vi "Module (Rename).vi"(8 "Error In":errorcluster) -> (0 "Last Error":errorcluster)   [LabVIEW 2015, in "Generic Module Library.lvlib" / "Template G_Module.lvlib"]
uses:
  Template G_Module.lvlib
  Module Class/Rename.lvclass
panel:
  in  "Stop":bool
  in  "Debug Toggle":bool
  in  "Debug Tab":T1(tab)
  out "Timing Target (ms)":i16
  out "Module Iterations":u64
  out "Last Executed Case":string
  in  "Configure":bool
  in  "View Log":bool
  in  "Ping":bool
  out "Ping Response":string
  out "Debug Log":string
  out "Received @":timestamp
  out "Current Error":errorcluster
  out "Received @":timestamp
  out "Received @":timestamp
  # ">>Newest>>"
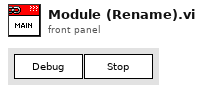
[diagram p1: front panel]
types:
  T1 = enum32{"Module Data/Commands", "Module Log", "Current Error", "Start Error", "Close Error"}
  T2 = typedef "Generic Module Library.lvlib/Template G_Module.lvlib/Broadcast List.ctl" = cluster{"Module Started":refnum<user-event>, "Module Error":refnum<user-event>, "Module Pong":refnum<user-event>, "Module Status":refnum<user-event>, "Module Stopping":refnum<user-event>, "Module Stopped":refnum<user-event>, "Module Reinitialized":refnum<user-event>}
  T3 = cluster{"Event Registration Refnum":refnum<event-registration>, "Stop Event Refnum":refnum<event-registration>}
  T4 = typedef "Generic Module Library.lvlib/Template G_Module.lvlib/Acknowledge Data Cluster.ctl" = cluster{"Ack Requested":bool, "Ack Notifier Ref":refnum<notifier>, "Response Payload":T5}
  T5 = typedef "Generic Module Library.lvlib/Template G_Module.lvlib/Ack Payload.ctl" = cluster{"Response Data":string, "error out":errorcluster}
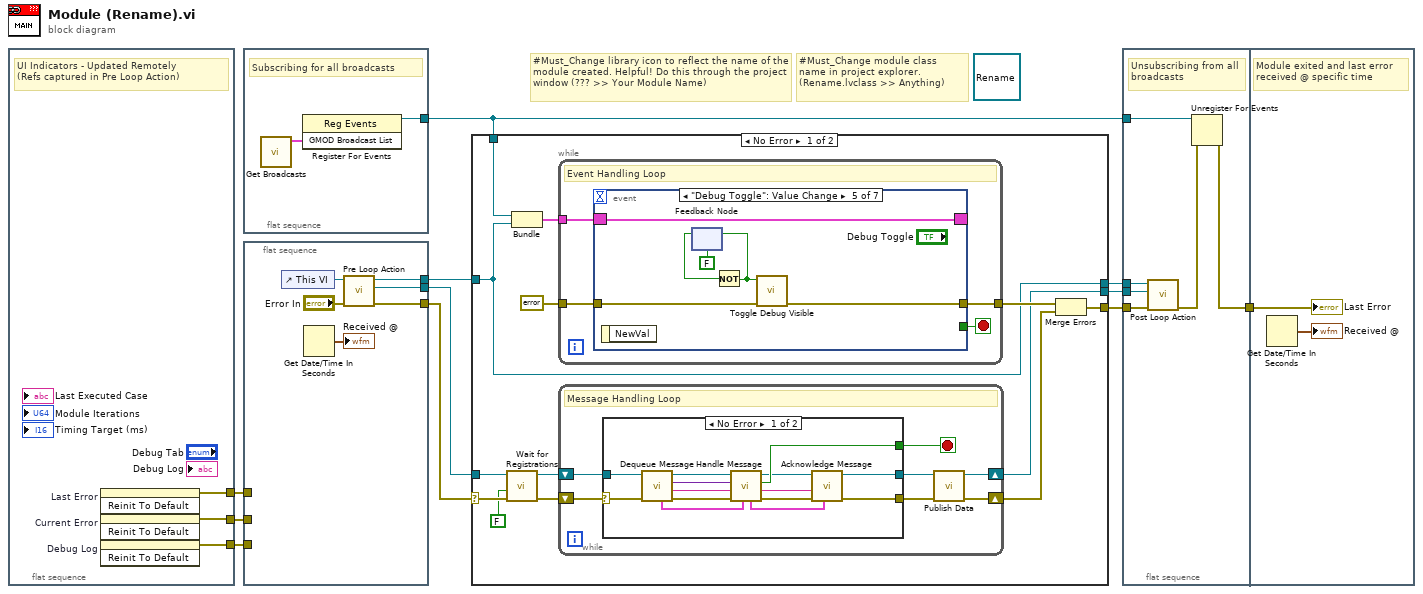
[diagram p0: block diagram]
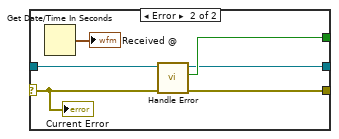
[diagram p2: hidden frame]
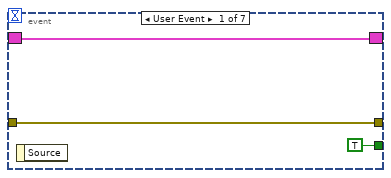
[diagram p3: hidden frame]
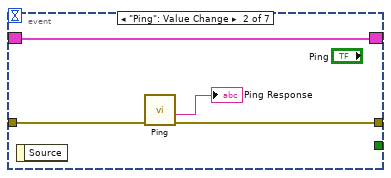
[diagram p4: hidden frame]
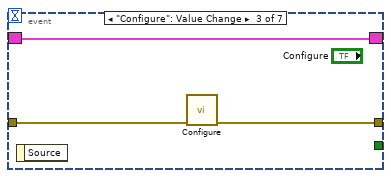
[diagram p5: hidden frame]
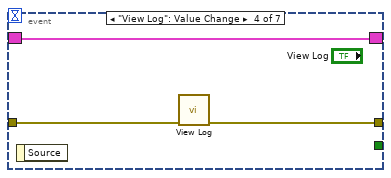
[diagram p6: hidden frame]
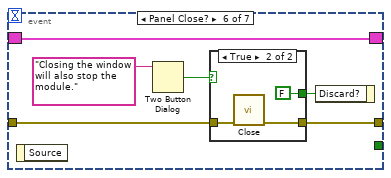
[diagram p7: hidden frame]
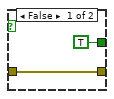
[diagram p8: hidden frame]
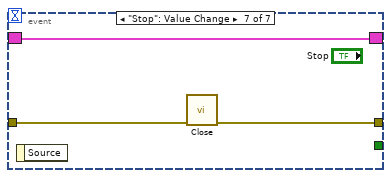
[diagram p9: hidden frame]
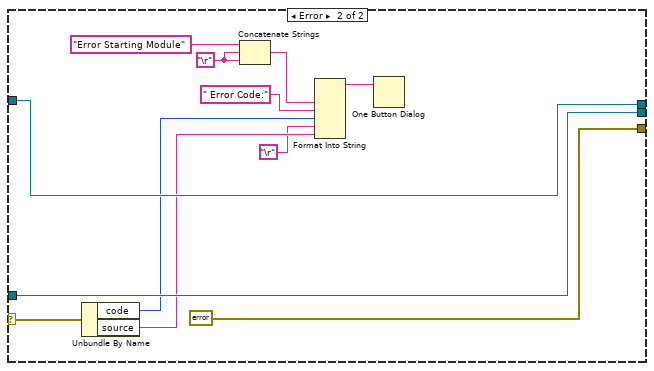
[diagram p10: hidden frame]
diagram:
  (unwired) refnum<class "Rename.lvclass"> refnum ("Generic Module Library.lvlib:Template G_Module.lvlib:Rename.lvclass")
  # "#Must_Change library icon to reflect the name of the module created. Helpful! Do this through the project window (??? >> Your Module Name)"
  # "#Must_Change module class name in project explorer. (Rename.lvclass >> Anything)"
  n1 = flat-sequence {
    tunnel: [w14] -> w5
    tunnel: [w13] -> w4
    tunnel: [w12] -> w3
    frame #0 {
      # "UI Indicators - Updated Remotely \n(Refs captured in Pre Loop Action)"
      n2 = invoke on="Last Error" class="Clust (strict)" method="Reinit To Default"() -> (error out=w14:errorcluster)  [unwired: 3 in, 2 out]
      n3 = invoke on="Current Error" class="Clust (strict)" method="Reinit To Default"() -> (error out=w13:errorcluster)  [unwired: 3 in, 2 out]
      n4 = invoke on="Debug Log" class="Str" method="Reinit To Default"() -> (error out=w12:errorcluster)  [unwired: 3 in, 2 out]
    }
  }
  n5 = flat-sequence {
    tunnel: [w15] -> w2
    frame #0 {
      # "Subscribing for all broadcasts"
      n6 = call "Get Broadcasts.vi"() -> ("GMOD Broadcast List"=w16:T2)  [unwired: 9 in, 2 out]
      n7 = register-events(w16) -> (reference out=w15:refnum<event-registration>)  [unwired: 2 in, 1 out]
    }
  }
  n8 = flat-sequence {
    tunnel: [w19] -> w11
    tunnel: [w18] -> w1
    tunnel: [w17] -> w6
    tunnel: w5 -> [_]
    tunnel: w4 -> [_]
    tunnel: w3 -> [_]
    frame #0 {
      n9 = control-ref of="This VI"() -> (w22:refnum<vi>)
      n10 = Get Date/Time In Seconds() -> (seconds since 1Jan1904=→"Received @":timestamp)
      n11 = call "Pre Loop Action.vi"("error in"="Error In", "Ref In"=w22) -> ("error out"=w17:errorcluster, "Module Data Out"=w19:refnum<class "Rename.lvclass">, "Stop Event Refnum"=w18:refnum<event-registration>)  [unwired: 7 in]
    }
  }
  n12 = case shown="No Error" w6 {
    selector: w6 -> [w27 w103]
    tunnel: w11 -> [w34 w111]
    tunnel: [w32 errorcluster {"status"=FALSE, "code"=0, "source"=""} ("error IO")] -> w9
    tunnel: [w31 w111] -> w8
    tunnel: [w23 w110] -> w7
    tunnel: w2 -> [w25 _]
    tunnel: w1 -> [w23 w110]
    frame No Error {
      n13 = call "Wait for Registrations.vi"("error in"=w27, "Wait for Reg Confirmation? (F)"=FALSE, "Module Data In"=w34) -> ("error out"=w29:errorcluster, "Module Data Out"=w30:refnum<class "Rename.lvclass">)  [unwired: 6 in, 1 out]
      n14 = Bundle("Event Registration Refnum"=w25, "Stop Event Refnum"=w23) -> (w24:T3)  [unwired: 1 in]
      n15 = while {
        tunnel: w24 -> [w64]
        tunnel: errorcluster {"status"=FALSE, "code"=0, "source"=""} ("error out") -> [w65]
        tunnel: [w66] -> w35
        stop <- w63 stop-if-true
        # "Event Handling Loop"
        n16 = event shown="[4] \"Debug Toggle\": Value Change" {
          selector: w64 -> [w67 w70 w76 w79 w85 w86 w99]
          dyn-events: [w67 w70 w76 w79 w85 w86 w99] -> _
          timeout: _ -> [_ _ _ _ _ _ _]
          tunnel: [w69 w72 w74 w77 w83 w89 w97] -> w66
          tunnel: w65 -> [w69 w73 w75 w78 w84 w90 w98]
          tunnel: [TRUE _ _ _ _ _ _] -> w63
          event User Event {
            n17 = event-data() -> ()  [unwired: 1 in, 1 out]
          }
          event "Ping": Value Change {
            n18 = event-data() -> ()  [unwired: 1 in, 1 out]
            n19 = call "Ping.vi"("error in"=w73) -> ("error out"=w72:errorcluster, "Response"=→"Ping Response":string)  [unwired: 8 in, 1 out]
          }
          event "Configure": Value Change {
            n20 = event-data() -> ()  [unwired: 1 in, 1 out]
            n21 = call "Configure.vi"("error in"=w75) -> ("error out"=w74:errorcluster)  [unwired: 10 in]
          }
          event "View Log": Value Change {
            n22 = event-data() -> ()  [unwired: 1 in, 1 out]
            n23 = call "View Log.vi"("error in"=w78) -> ("error out"=w77:errorcluster)  [unwired: 10 in]
          }
          event "Debug Toggle": Value Change {
            n24 = event-data() -> ()  [unwired: 1 in, 1 out]
            n25 = feedback #1(FALSE) -> (w81:bool)
            n26 = Not(x=w81) -> (.not. x?=w82:bool)
            n27 = feedback-in #1(w82) -> ()
            n28 = call "Toggle Debug Visible.vi"("error in"=w84, "Visible?"=w82) -> ("error out"=w83:errorcluster)  [unwired: 9 in]
          }
          event Panel Close? {
            n29 = event-data() -> ()  [unwired: 1 in, 1 out]
            n30 = Two Button Dialog(message="Closing the window will also stop the module.") -> (T button?=w87:bool)  [unwired: 2 in]
            n31 = case shown="True" w87 {
              tunnel: [TRUE ("Discard?") FALSE ("Discard?")] -> w91
              tunnel: w90 -> [w92 w95]
              tunnel: [w92 w94] -> w89
              frame False {
              }
              frame True {
                n32 = call "Close.vi"("error in"=w95) -> ("error out"=w94:errorcluster)  [unwired: 9 in, 1 out]
              }
            }
            n33 = event-data("Discard?"=w91) -> ()  [unwired: 1 in, 1 out]
          }
          event "Stop": Value Change {
            n34 = event-data() -> ()  [unwired: 1 in, 1 out]
            n35 = call "Close.vi"("error in"=w98) -> ("error out"=w97:errorcluster)  [unwired: 9 in, 1 out]
          }
        }
      }
      n36 = while {
        shift-right: [w36] -> w31
        shift-left: w30 -> [w41]
        shift-right: [w37] -> w33
        shift-left: w29 -> [w40]
        stop <- w42 stop-if-true
        # "Message Handling Loop"
        n37 = case shown="No Error" w40 {
          selector: w40 -> [w55 w57]
          tunnel: [w50 w62] -> w42
          tunnel: [w54 w61] -> w39
          tunnel: [w53 w60] -> w38
          tunnel: w41 -> [w56 w59]
          frame No Error {
            n38 = call "Dequeue Message.vi"("error in"=w55, "Module Data In"=w56) -> ("error out"=w46:errorcluster, "Module Action"=w45:string, "Message Data"=w44:variant, "Module Data Out"=w43:refnum<class "Rename.lvclass">, "Acknowledge Data"=w47:T4)  [unwired: 5 in]
            n39 = call "Handle Message.vi"("Acknowledge Data"=w47, "error in (no error)"=w46, "Module Action"=w45, "Message Data Out"=w44, "Module Data In"=w43) -> ("error out"=w52:errorcluster, "Module Action"=w51:string, "Stop Module"=w50:bool, "Module Data Out"=w49:refnum<class "Rename.lvclass">, "Acknowledge Data"=w48:T4)  [unwired: 2 in]
            n40 = call "Acknowledge Message.vi"("Acknowledge Data"=w48, "error in"=w52, "Module Action"=w51, "Module Data In"=w49) -> ("error out"=w54:errorcluster, "Module Data Out"=w53:refnum<class "Rename.lvclass">)  [unwired: 6 in]
          }
          frame Error {
            n41 = Get Date/Time In Seconds() -> (seconds since 1Jan1904=→"Received @":timestamp)
            n42 = call "Handle Error.vi"("error in (no error)"=w57, "Rename in"=w59) -> ("error out"=w61:errorcluster, "Stop Module"=w62:bool, "Rename out"=w60:refnum<class "Rename.lvclass">)  [unwired: 7 in]
            "Current Error" <- w57
          }
        }
        n43 = call "Publish Data.vi"("error passthrough"=w39, "Module Data In"=w38) -> ("error passthrough"=w37:errorcluster, "Module Data Out"=w36:refnum<class "Rename.lvclass">)  [unwired: 8 in]
      }
      n44 = Merge Errors(w35, w33) -> (w32:errorcluster)
    }
    frame Error {
      w108 = "\r"
      n45 = Unbundle By Name(w103) -> ("code"=w107:i32, "source"=w105:string)
      n46 = Concatenate Strings("Error Starting Module" ("string"), w108, w108) -> (w101:string)
      n47 = Format Into String(w101, " Error Code:" ("input 2"), w107, "\r", w105) -> (resulting string=w100:string)  [unwired: 3 in, 1 out]
      n48 = One Button Dialog(message=w100) -> ()  [unwired: 1 in, 1 out]
    }
  }
  n49 = flat-sequence {
    tunnel: w9 -> [w117]
    tunnel: w8 -> [w116]
    tunnel: w2 -> [w115]
    tunnel: w7 -> [w114]
    tunnel: [w112] -> w10
    tunnel: w10 -> [w118]
    frame #0 {
      # "Unsubscribing from all broadcasts"
      n50 = call "Post Loop Action.vi"("error in (no error)"=w117, "Module Data In"=w116, "Event Registration Refnum"=w114) -> ("error out"=w113:errorcluster)  [unwired: 8 in]
      n51 = Unregister For Events(event registration refnum=w115, error in=w113) -> (error out=w112:errorcluster)
    }
    frame #1 {
      # "Module exited and last error received @ specific time"
      n52 = Get Date/Time In Seconds() -> (seconds since 1Jan1904=→"Received @":timestamp)
      "Last Error" <- w118
    }
  }
